vi "Panel Request In Editabled State.vi"(8 "error in (no error)":errorcluster, 10 "Panel Behavior(class)":refnum<class "Panel Behavior.lvclass">, 11 "EditPanel in":refnum<class "EditPanel API.lvclass">) -> (0 "error out":errorcluster, 3 "EditPanel out":refnum<class "EditPanel API.lvclass">)   [LabVIEW 2015, in "EditPanel API.lvlib" / "EditPanel API.lvclass"]
uses:
  EditPanel API.lvclass
  Panel Request/Panle Requeset Behavior/Panel Behavior.lvclass
  EditPanel API.lvclass/EditPanel API.ctl
  Console Reply/Console Reply/Console Reply.lvclass/Console Reply.ctl
  Panel Request/Panel Request Msg/Panel Request Msg.lvclass/Panel Request Msg.ctl
  <vilib>/ActorFramework/Message Enqueuer/Message Enqueuer.lvclass/Message Enqueuer.ctl
  <vilib>/ActorFramework/Message Enqueuer/Enqueue.vi
  <vilib>/ActorFramework/Message Priority Queue/Priority Enqueue.vi
  <vilib>/ActorFramework/Message Enqueuer/Message Enqueuer.lvclass
  Panel Request/Panel Request Msg/Panel Request Msg.lvclass
  Console Reply/Console Reply/Console Reply.lvclass
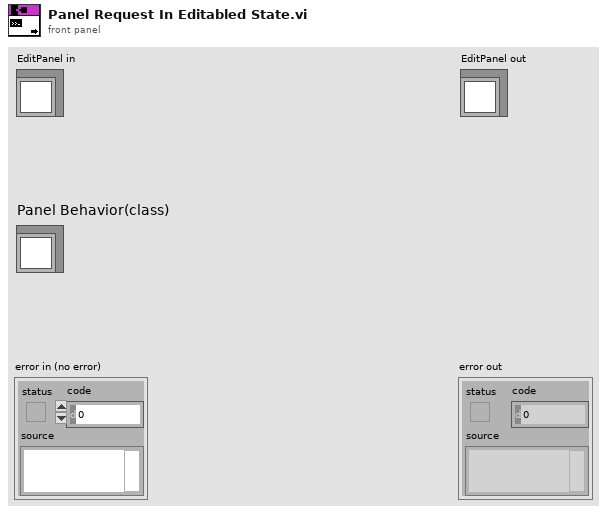
[diagram p1: front panel]
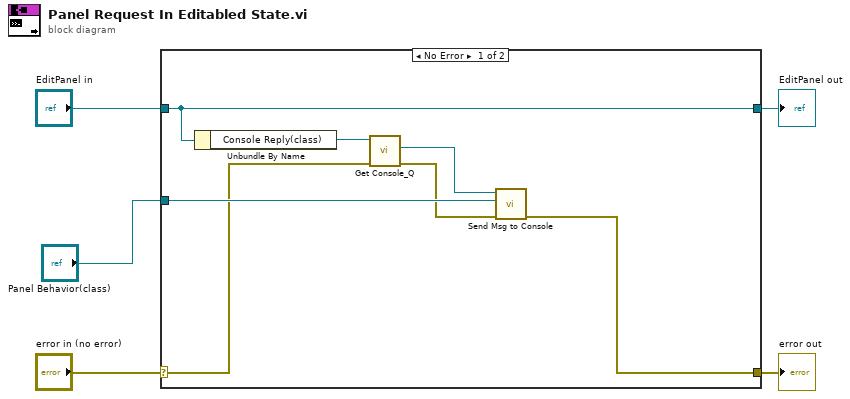
[diagram p0: block diagram]
diagram:
  n1 = case shown="No Error" "error in (no error)" {
    selector: "error in (no error)" -> [w7 w14]
    tunnel: [w11 w14] -> w4
    tunnel: [w12 w13] -> w2
    tunnel: "EditPanel in" -> [w12 w13]
    tunnel: "Panel Behavior(class)" -> [w10 _]
    frame No Error {
      n2 = Unbundle By Name(w12) -> ("Console Reply(class)"=w9:refnum<class "Console Reply.lvclass">)
      n3 = call "Get Console_Q.vi"("error in (no error)"=w7, "Console Reply.lvclass"=w9) -> ("error out"=w6:errorcluster, "Console Q"=w8:refnum<class "Message Enqueuer.lvclass">)  [unwired: 7 in, 1 out]
      n4 = call "Send Msg to Console.vi"("error in (no error)"=w6, "Panel Behavior.lvclass"=w10, "Message Enqueuer"=w8) -> ("error out"=w11:errorcluster)  [unwired: 7 in, 1 out]
    }
    frame Error {
    }
  }
  "error out" <- w4
  "EditPanel out" <- w2
